vi "Global control type freno.vi"() -> ()   [LabVIEW 2019]
panel:
  in  "Value":T1(ring)
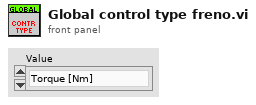
[diagram p1: front panel]
types:
  T1 = enum32{"Torque [Nm]", "Power [W]", "Speed [RPM]", "Corrente [A]"}
diagram:
